vi "Stop Core.vi"(10 "final error code":i32, 11 "DAQ Actor (Slave) in":refnum<class "DAQ Actor (Slave).lvclass">) -> (3 "DAQ Actor (Slave) out":refnum<class "DAQ Actor (Slave).lvclass">)   [LabVIEW 2012, in "Data Acquisition.lvlib" / "DAQ Actor (Slave).lvclass"]
doc: "(<B>Filename</B>: Actor Framework.lvlib:Actor.lvclass:Stop Core.vi)\n\nDefines what the actor does before it stops. Use the <B>final error code</B> input to determine whether the actor shut down in response to an error.\n\nBy default, this method does nothing. A descendant class may override it to define behavior, such as shutting down any processes the actor initiated in its override of the Actor Core method."
uses:
  DAQ Actor (Slave).lvclass
  Class DAQ Actor/DAQ Actor.lvclass
  DAQ Actor (Slave).lvclass/DAQ Actor (Slave).ctl
  <vilib>/ActorFramework/Stop Msg/Stop Msg.lvclass/Stop Msg.ctl
  <vilib>/ActorFramework/Message Enqueuer/Message Enqueuer.lvclass/Message Enqueuer.ctl
  <vilib>/ActorFramework/Stop Msg/Send Emergency Stop.vi
  <vilib>/ActorFramework/Stop Msg/Send Normal Stop.vi
  <vilib>/ActorFramework/Message Enqueuer/Enqueue Critical.vi
  <vilib>/ActorFramework/Message Enqueuer/Enqueue.vi
  <vilib>/ActorFramework/Message Priority Queue/Priority Enqueue.vi
  <vilib>/ActorFramework/Stop Msg/Stop Msg.lvclass
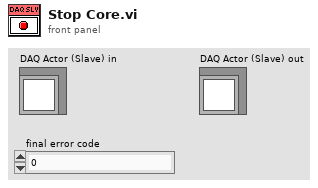
[diagram p1: front panel]
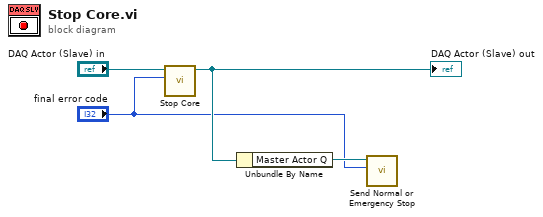
[diagram p0: block diagram]
diagram:
  n1 = call-parent "Stop Core.vi"("final error code"="final error code", "DAQ Actor in"="DAQ Actor (Slave) in") -> ("DAQ Actor out"=w3:refnum<class "DAQ Actor (Slave).lvclass">)  [unwired: 9 in]
  "DAQ Actor (Slave) out" <- w3
  n2 = Unbundle By Name(w3) -> ("Master Actor Q"=w2:refnum<class "Message Enqueuer.lvclass">)
  n3 = call <vilib>:"Send Normal or Emergency Stop.vi"("final error code"="final error code", "Message Enqueuer"=w2) -> ()  [unwired: 9 in, 1 out]
